vi "Dilate_Low_Manual.vi"(4 "Error IN Toolkit":i32, 5 "Error IN LabVIEW":errorcluster, 6 "Radio":i32, 8 "Blocks":i32, 10 "Threads":i32) -> (18 "Error OUT Toolkit":i32, 19 "Error OUT LabVIEW":errorcluster)   [LabVIEW 2018]
doc: "\"Dilate\" is the opposite of \"Erode\". Here, a pixel element is '1' if at least one pixel of the image of those falling inside the kernel (radio) window is '1'. Therefore, Dilate increases the size of the foreground objects, that is, the white region. It receives the number of threads and blocks for the GPU and the radio known as the kernel, which is the checking area.\n\nFor correct operation it should receive an error that comes from a VI of some processing algorithm or that contains a copy data of CPU-GPU."
uses:
  dll/LibreriaAutis_3.dll
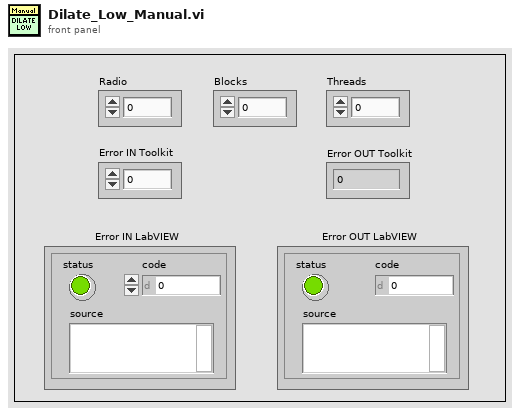
[diagram p1: front panel]
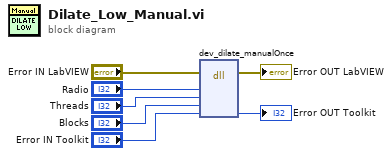
[diagram p0: block diagram]
diagram:
  n1 = dll-call lib="C:/Users/AUTIS/Desktop/LibreriaAUTIS/LabVIEW/dll/LibreriaAutis_3.dll" fn="dev_dilate_manualOnce"(error in="Error IN LabVIEW", "radio"="Radio", "threads"="Threads", "blocks"="Blocks", "error"="Error IN Toolkit") -> (error out=→"Error OUT LabVIEW":errorcluster, "error"=→"Error OUT Toolkit":i32)  [unwired: 6 in, 1 out]
